vi "Simple_LV2.vi"(0 "Data_In":dbl format="%#_13g", 11 "Error_In":errorcluster, 13 "Operation":T1=enum."Read") -> (4 "Data_Out":dbl format="%#_13g", 15 "Error_Out":errorcluster)   [LabVIEW 2021]
doc: "This a simply LV2 which can be write and read accross VIs"
uses:
  Controls/Operation_Simple_LV2.ctl
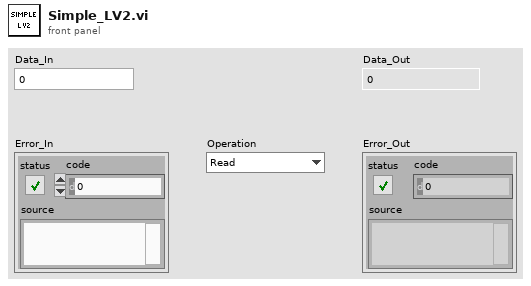
[diagram p1: front panel]
types:
  T1 = typedef "Operation_Simple_LV2.ctl" = enum16{"Write", "Read"}
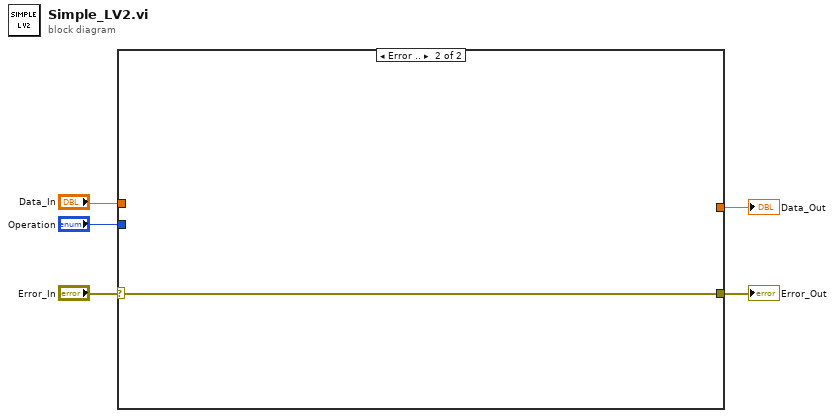
[diagram p0: block diagram]
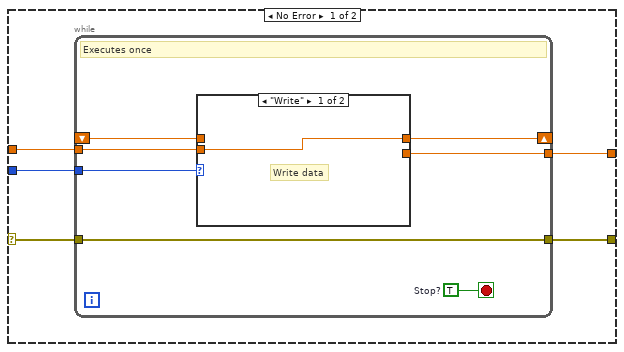
[diagram p2: hidden frame]
diagram:
  n1 = case shown="Error .." "Error_In" {
    selector: "Error_In" -> [w6 w20]
    tunnel: "Operation" -> [w10 _]
    tunnel: [w9 w20] -> w4
    tunnel: "Data_In" -> [w8 _]
    tunnel: [w7 _] -> w2
    frame No Error {
      n2 = while {
        shift-right: [w17] -> _
        shift-left: _ -> [w16]
        tunnel: w10 -> [w15]
        tunnel: w8 -> [w12]
        tunnel: [w11] -> w7
        tunnel: w6 -> [w13]
        tunnel: [w13] -> w9
        stop <- w14 stop-if-true
        w14 = TRUE  # Stop?
        # "Executes once"
        n3 = case shown="\"Write\"" w15 {
          tunnel: [w18 w19] -> w17
          tunnel: w16 -> [_ w19]
          tunnel: w12 -> [w18 _]
          tunnel: [_ w19] -> w11
          frame "Write" {
            # "Write data"
          }
          frame "Read" {
            # "Read data"
          }
        }
      }
    }
    frame Error {
    }
  }
  "Error_Out" <- w4
  "Data_Out" <- w2
